vi "Automation Update Test Name.vi"(8 "error in":errorcluster, 10 "Test Name":string, 11 "Base Software in":refnum<class "Main.lvclass">) -> (0 "error out":errorcluster, 3 "Base Software out":refnum<class "Main.lvclass">)   [LabVIEW 2023, in "Main.lvlib" / "Main.lvclass"]
uses:
  Project/Main.lvclass
  builds/Engine/Engine.lvlibp/Project/Engine.lvclass
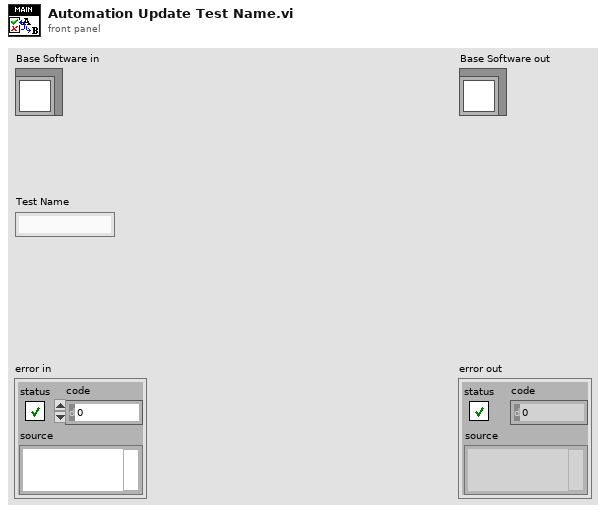
[diagram p1: front panel]
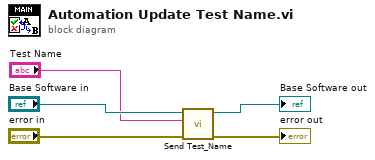
[diagram p0: block diagram]
diagram:
  n1 = call "Send Test_Name.vi"("error in"="error in", "Test Name"="Test Name", "Engine in"="Base Software in") -> ("error out"=→"error out":errorcluster, "Engine out"=→"Base Software out":refnum<class "Main.lvclass">)  [unwired: 7 in]
